vi "Non-Linearity.vi"(10 "Hall-Effect":dbl[](array[numeric]), 11 "Encoder":dbl[](array[numeric])) -> (2 "Non-Linearity (%)":dbl, 3 "Best Linear Fit":dbl[](array[numeric]))   [LabVIEW 2019]
uses:
  <vilib>/Analysis/NI_AALPro.lvlib
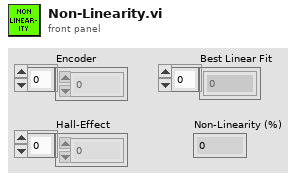
[diagram p1: front panel]
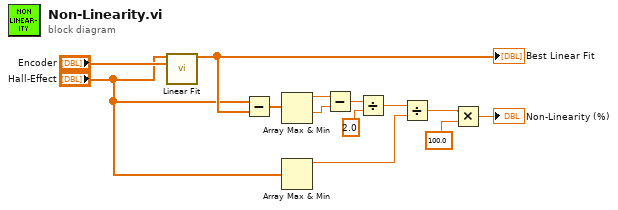
[diagram p0: block diagram]
diagram:
  n1 = call <vilib>:"Linear Fit.vi"("Y"="Hall-Effect", "X"="Encoder") -> ("Best Linear Fit"=w8:dbl[])  [unwired: 9 in, 4 out]
  "Best Linear Fit" <- w8
  n2 = Subtract(x="Hall-Effect", y=w8) -> (x-y=w9:dbl[])
  n3 = Array Max & Min(array=w9) -> (max value=w10:dbl, min value=w11:dbl)  [unwired: 2 out]
  n4 = Array Max & Min(array="Hall-Effect") -> (max value=w5:dbl)  [unwired: 3 out]
  n5 = Subtract(x=w10, y=w11) -> (x-y=w12:dbl)
  n6 = Divide(x=w12, y=2.0) -> (x/y=w6:dbl)
  n7 = Divide(x=w6, y=w5) -> (x/y=w4:dbl)
  n8 = Multiply(x=w4, y=100.0) -> (x*y=→"Non-Linearity (%)":dbl)
